vi "niDTS WLAN Dut Tx Configure.vi"(0 "Dut Handle in":T6, 5 "niDTS WLAN DUT Parameters":T1={"WLAN Type"=enum."n - MCS7", "Bandwidth (Hz)"=enum."20 MHz", "Channel"=36, "Guard Interval"=enum."SHORT", "FEC Coding"=enum."LDPC", "Power (dBm)"=0.0, "Payload Length (bytes)"=1500, "16 Symbols"=TRUE, "Chains"=[TRUE, FALSE, FALSE, FALSE]}, 7 "Apply Additional Defaults":bool=TRUE, 11 "error in (no error)":errorcluster) -> (4 "Dut Handle":T6, 15 "error out":errorcluster)   [LabVIEW 2015, in "niDTS WLAN.lvlib"]
doc: "Set the basic parameters for the WLAN TX Test. \n\nInputs:\n* Apply Additional Defaults. This allows more advanced parameters, which are dependant on the inputs, to have their default values set.\n\nCallbacks:\n* WLAN DUT Additional Defaults\n\nNote: This behavior is expected to be depricated when full parameter sets are passed as inputs and the input dependant defaults are calculated on the top parameter setting level."
uses:
  niDTS WLAN.lvlib
  Framework/Dut/Includes/niDTS Dut INC Handle.ctl
  Framework/Dut/Objects/BASE_class/niDTS Dut.lvclass
  Includes/niDTS WLAN DUT INC Parameters.ctl
  Includes/niDTS WLAN INC Type.ctl
  Includes/niDTS WLAN INC CH BW.ctl
  Includes/niDTS WLAN INC GI.ctl
  Includes/niDTS WLAN INC FEC Coding.ctl
  Includes/niDTS WLAN Dut INC Handle.ctl
  Objects/BASE_class/niDTS WLAN Dut.lvclass
  Objects/niDTS WLAN Dut Data/niDTS WLAN Dut Data.lvclass
  Framework/Logger/Objects/BASE_class/niDTS Logger.lvclass
  Framework/niDTS Framework.lvlib
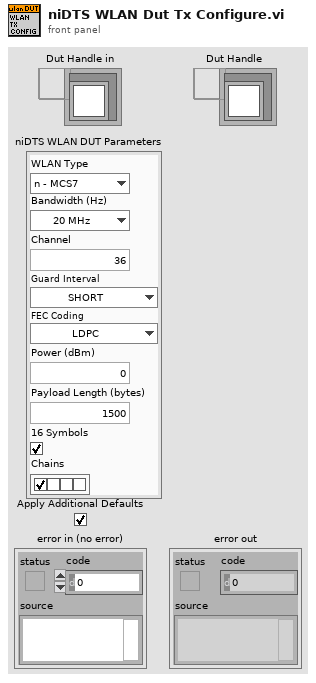
[diagram p1: front panel]
types:
  T1 = typedef "niDTS WLAN.lvlib/niDTS WLAN DUT INC Parameters.ctl" = cluster{"WLAN Type":T2, "Bandwidth (Hz)":T3, "Channel":i32, "Guard Interval":T4, "FEC Coding":T5, "Power (dBm)":dbl, "Payload Length (bytes)":i32, "16 Symbols":bool, "Chains":bool[]}
  T2 = typedef "niDTS WLAN.lvlib/niDTS WLAN INC Type.ctl" = enum16{"b - 1 Mbps", "b - 2 Mbps", "b - 5.5 Mbps", "b - 11 Mbps", "ag - 6 Mbps", "ag - 9 Mbps", "ag - 12 Mbps", "ag - 18 Mbps", "ag - 24 Mbps", "ag - 36 Mbps", "ag - 48 Mbps", "ag - 54 Mbps", "n - MCS0", "n - MCS1", "n - MCS2", "n - MCS3", "n - MCS4", "n - MCS5", "n - MCS6", "n - MCS7", "n - MCS8", "n - MCS9", "n - MCS10", "n - MCS11", "n - MCS12", "n - MCS13", "n - MCS14", "n - MCS15", "n - MCS16", "n - MCS17", "n - MCS18", "n - MCS19", "n - MCS20", "n - MCS21", "n - MCS22", "n - MCS23", "n - MCS24", "n - MCS25", "n - MCS26", "n - MCS27", "n - MCS28", "n - MCS29", "n - MCS30", "n - MCS31", "ac - MCS0 -1", "ac - MCS1 -1", "ac - MCS2 -1", "ac - MCS3 -1", "ac - MCS4 -1", "ac - MCS5 -1", "ac - MCS6 -1", "ac - MCS7 -1", "ac - MCS8 -1", "ac - MCS9 -1", "ac - MCS0 -2", "ac - MCS1 -2", "ac - MCS2 -2", "ac - MCS3 -2", "ac - MCS4 -2", "ac - MCS5 -2", "ac - MCS6 -2", "ac - MCS7 -2", "ac - MCS8 -2", "ac - MCS9 -2", "ac - MCS0 -3", "ac - MCS1 -3", "ac - MCS2 -3", "ac - MCS3 -3", "ac - MCS4 -3", "ac - MCS5 -3", "ac - MCS6 -3", "ac - MCS7 -3", "ac - MCS8 -3", "ac - MCS9 -3", "ac - MCS0 -4", "ac - MCS1 -4", "ac - MCS2 -4", "ac - MCS3 -4", "ac - MCS4 -4", "ac - MCS5 -4", "ac - MCS6 -4", "ac - MCS7 -4", "ac - MCS8 -4", "ac - MCS9 -4"}
  T3 = typedef "niDTS WLAN.lvlib/niDTS WLAN INC CH BW.ctl" = enum16{"20 MHz", "40 MHz", "80 MHz", "160 MHz"}
  T4 = typedef "niDTS WLAN.lvlib/niDTS WLAN INC GI.ctl" = enum16{"LONG", "SHORT"}
  T5 = typedef "niDTS WLAN.lvlib/niDTS WLAN INC FEC Coding.ctl" = enum16{"BCC", "LDPC"}
  T6 = typedef "niDTS Framework.lvlib/niDTS Dut INC Handle.ctl" = refnum<data-value>
  T7 = typedef "niDTS WLAN.lvlib/niDTS WLAN Dut INC Handle.ctl" = refnum<data-value>
  T8 = typedef "niDTS Framework.lvlib/niDTS Logger INC Handle.ctl" = refnum<data-value>
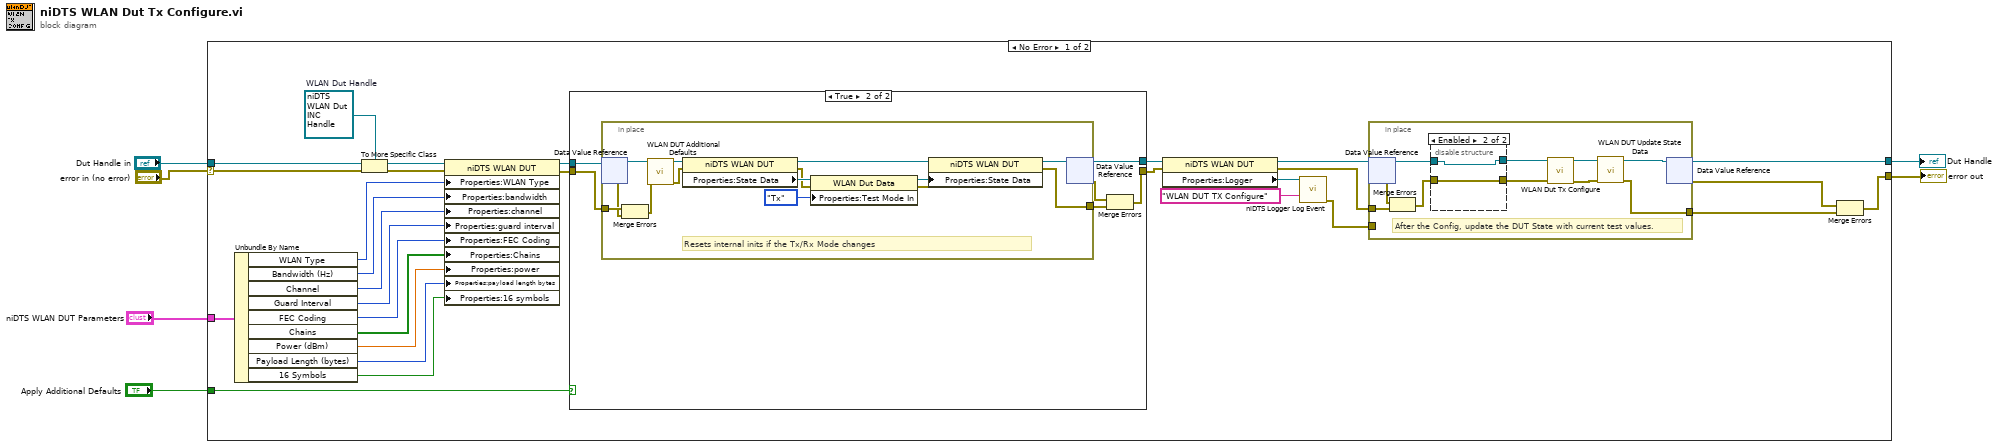
[diagram p0: block diagram]
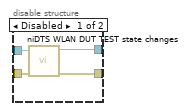
[diagram p2: hidden frame]
diagram:
  n1 = case shown="No Error" "error in (no error)" {
    selector: "error in (no error)" -> [w23 w74]
    tunnel: "Dut Handle in" -> [w35 w75]
    tunnel: "niDTS WLAN DUT Parameters" -> [w31 _]
    tunnel: "Apply Additional Defaults" -> [w26 _]
    tunnel: [w22 w75] -> w3
    tunnel: [w19 w74] -> w2
    frame No Error {
      w34 = T7 refnum  # WLAN Dut Handle
      n2 = Unbundle By Name(w31) -> ("WLAN Type"=w30:T2, "Bandwidth (Hz)"=w29:T3, "Channel"=w28:i32, "Guard Interval"=w27:T4, "FEC Coding"=w7:T5, "Chains"=w9:bool[], "Power (dBm)"=w18:dbl, "Payload Length (bytes)"=w10:i32, "16 Symbols"=w8:bool)
      n3 = To More Specific Class(target class=w34, reference=w35, error in=w23) -> (specific class reference=w33:T7, error out=w32:errorcluster)
      n4 = property class="niDTS WLAN DUT"(reference=w33, error in=w32, "Properties:WLAN Type"=w30, "Properties:bandwidth"=w29, "Properties:channel"=w28, "Properties:guard interval"=w27, "Properties:FEC Coding"=w7, "Properties:Chains"=w9, "Properties:power"=w18, "Properties:payload length bytes"=w10, "Properties:16 symbols"=w8) -> (reference out=w25:T7, error out=w24:errorcluster)
      n5 = case shown="True" w26 {
        tunnel: w25 -> [w53 w59]
        tunnel: w24 -> [w52 w58]
        tunnel: [w53 w56] -> w17
        tunnel: [w52 w55] -> w16
        frame False {
        }
        frame True {
          n6 = in-place {
            in-place-border: w58 -> [w71]
            in-place-border: [w60] -> w54
            # "Resets internal inits if the Tx/Rx Mode changes"
            n7 = in-place-dvr #1(w59) -> (w73:refnum<class "niDTS WLAN Dut.lvclass">, w69:errorcluster)
            n8 = Merge Errors(w71, w69) -> (w70:errorcluster)
            n9 = call-dynamic "WLAN DUT Additional Defaults.vi"("niDTS WLAN DUT in"=w73, "error in (no error)"=w70) -> ("niDTS WLAN DUT out"=w72:refnum<class "niDTS WLAN Dut.lvclass">, "error out"=w67:errorcluster)  [unwired: 12 in]
            n10 = property class="niDTS WLAN DUT"(reference=w72, error in=w67) -> (reference out=w68:refnum<class "niDTS WLAN Dut.lvclass">, error out=w64:errorcluster, "Properties:State Data"=w65:refnum<class "niDTS WLAN Dut Data.lvclass">)
            n11 = property class="WLAN Dut Data"(reference=w65, error in=w64, "Properties:Test Mode In"=enum16{"Tx", "Rx"}."Tx" ("Test Mode In")) -> (reference out=w62:refnum<class "niDTS WLAN Dut Data.lvclass">, error out=w63:errorcluster)
            n12 = property class="niDTS WLAN DUT"(reference=w68, error in=w63, "Properties:State Data"=w62) -> (reference out=w66:refnum<class "niDTS WLAN Dut.lvclass">, error out=w60:errorcluster)
            n13 = in-place-dvr #1(w66) -> (w56:T7, w57:errorcluster)
          }
          n14 = Merge Errors(w57, w54) -> (w55:errorcluster)
        }
      }
      n15 = property class="niDTS WLAN DUT"(reference=w17, error in=w16) -> (reference out=w13:T7, error out=w12:errorcluster, "Properties:Logger"=w15:T8)
      n16 = call "niDTS Logger Log Event.vi"("Logger Handle"=w15, "Source/Location"="WLAN DUT TX Configure") -> ("error out"=w11:errorcluster)  [unwired: 11 in, 2 out]
      n17 = in-place {
        in-place-border: w12 -> [w45]
        in-place-border: [w40] -> w21
        in-place-border: w11 -> [_]
        # "After the Config, update the DUT State with current test values."
        n18 = in-place-dvr #2(w13) -> (w39:refnum<class "niDTS WLAN Dut.lvclass">, w44:errorcluster)
        n19 = Merge Errors(w44, w45) -> (w37:errorcluster)
        n20 = disable-structure shown="Enabled" {
          disable-tunnel: w39 -> [w49 w51]
          disable-tunnel: [w48 w51] -> w38
          disable-tunnel: w37 -> [w47 w50]
          disable-tunnel: [w46 w50] -> w36
          frame Disabled {
            n21 = call-dynamic "niDTS WLAN DUT TEST state changes.vi"("error in (no error)"=w47, "niDTS WLAN DUT in"=w49) -> ("error out"=w46:errorcluster, "niDTS WLAN DUT out"=w48:refnum<class "niDTS WLAN Dut.lvclass">)  [unwired: 8 in]
          }
          frame Enabled {
          }
        }
        n22 = call-dynamic "WLAN Dut Tx Configure.vi"("niDTS WLAN DUT in"=w38, "error in (no error)"=w36) -> ("niDTS WLAN DUT out"=w43:refnum<class "niDTS WLAN Dut.lvclass">, "error out"=w41:errorcluster)  [unwired: 12 in]
        n23 = call-dynamic "WLAN DUT Update State Data.vi"("error in (no error)"=w41, "niDTS WLAN DUT in"=w43) -> ("error out"=w40:errorcluster, "niDTS WLAN DUT out"=w42:refnum<class "niDTS WLAN Dut.lvclass">)  [unwired: 8 in]
        n24 = in-place-dvr #2(w42) -> (w22:T7, w20:errorcluster)
      }
      n25 = Merge Errors(w20, w21) -> (w19:errorcluster)
    }
    frame Error {
    }
  }
  "error out" <- w2
  "Dut Handle" <- w3
